vi "Wait at Rendezvous.vi"(4 "error in (no error)":errorcluster, 5 "ms timeout (-1)":i32=-1, 7 "rendezvous":T1) -> (0 "error out":errorcluster, 1 "timed out":bool, 3 "rendezvous out":T1)   [LabVIEW 2010]
doc: "Waits until a sufficient number of tasks have arrived at the rendezvous."
uses:
  RendezvousDataCluster.ctl
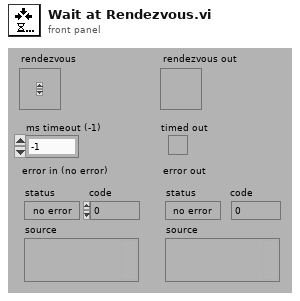
[diagram p1: front panel]
types:
  T1 = typedef "Rendezvous RefNum" = refnum<k1>
  T2 = typedef "RendezvousDataCluster.ctl" = cluster{"Threshold":i32, "Messenger Queues":refnum<queue>[]}
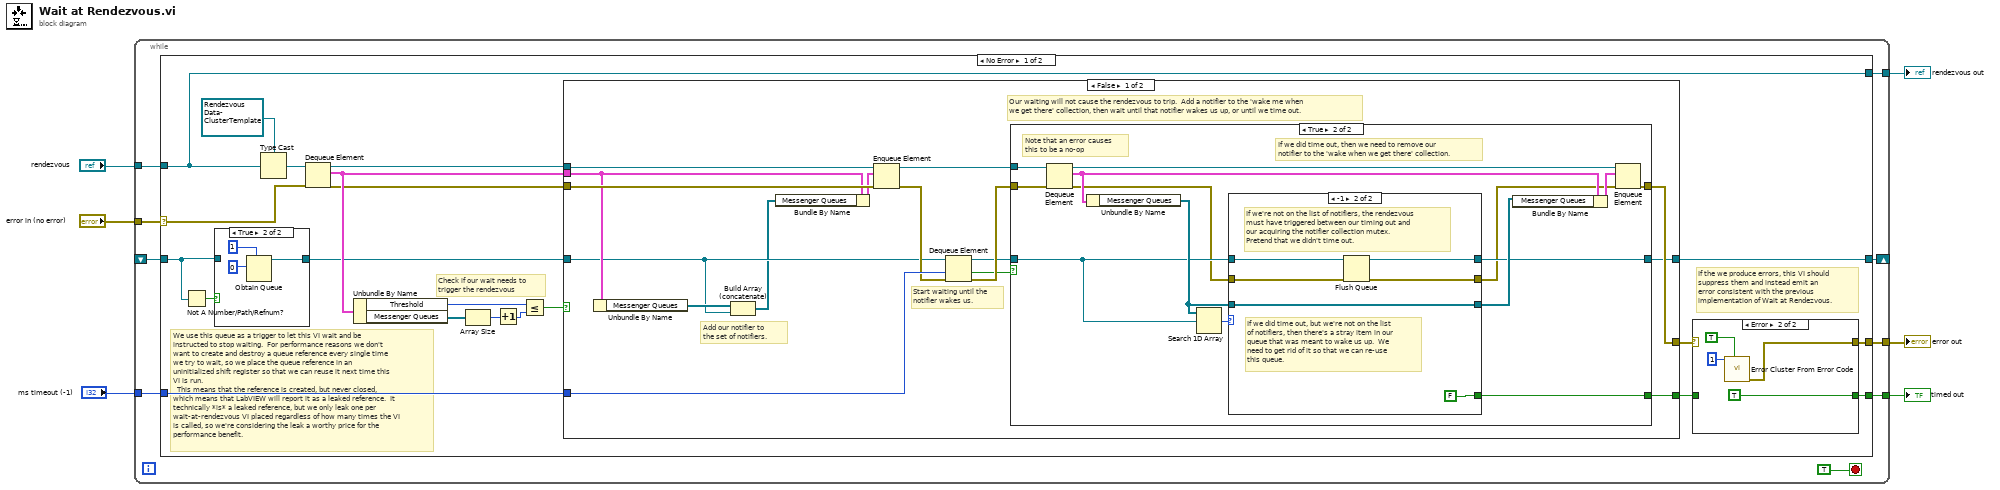
[diagram p0: block diagram]
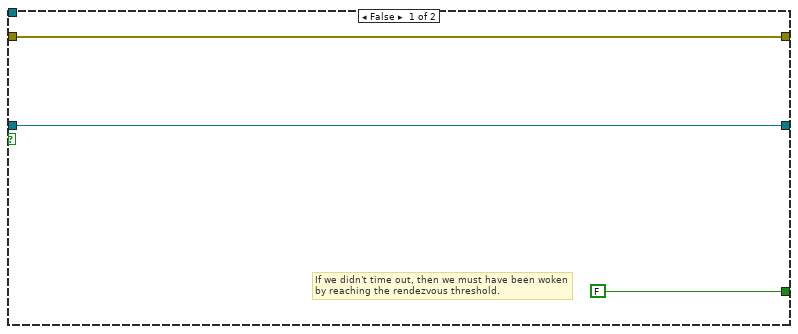
[diagram p3: hidden frame]
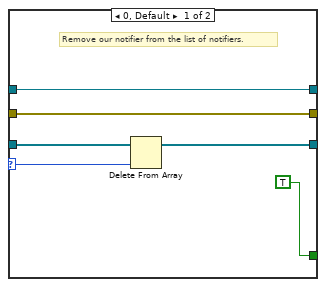
[diagram p4: hidden frame]
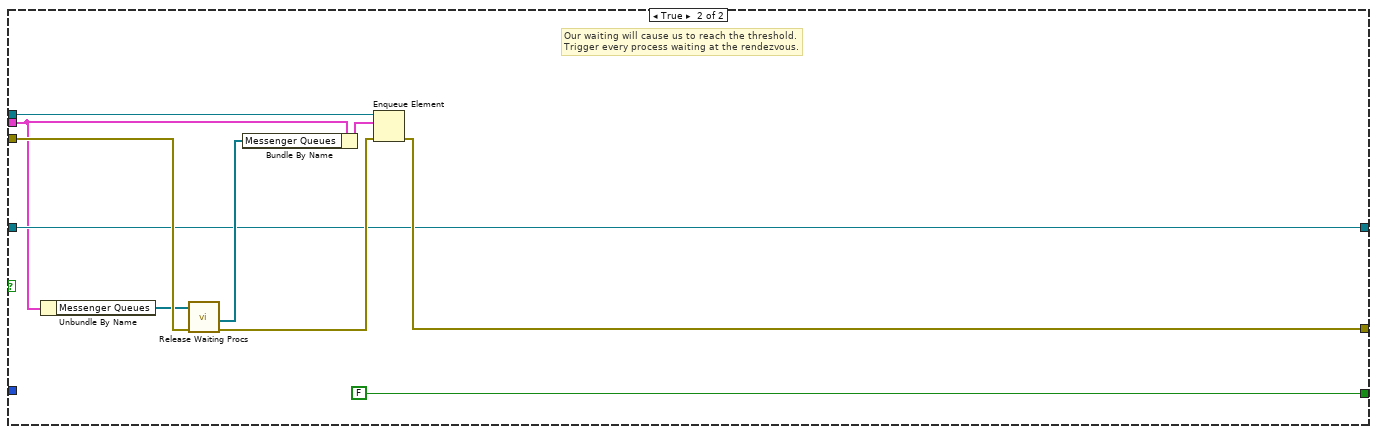
[diagram p5: hidden frame]
diagram:
  n1 = while {
    tunnel: [w15] -> w6
    tunnel: [w14] -> w5
    tunnel: "rendezvous" -> [w13]
    tunnel: [w12] -> w3
    tunnel: "error in (no error)" -> [w11]
    tunnel: "ms timeout (-1)" -> [w10]
    shift-right: [w8] -> _
    shift-left: _ -> [w7]
    stop <- TRUE stop-if-true
    n2 = case shown="No Error" w11 {
      selector: w11 -> [w23 w105]
      tunnel: [w36 w105] -> w15
      tunnel: [w35 FALSE] -> w14
      tunnel: w13 -> [w21 w104]
      tunnel: [w21 w104] -> w12
      tunnel: w10 -> [w29 _]
      tunnel: [w20 w102] -> w8
      tunnel: w7 -> [w17 w102]
      frame No Error {
        # "We use this queue as a trigger to let this VI wait and be instructed to stop waiting.  For performance reasons we don't want to create and destroy a queue reference every single time we try to wait, so we place the queue reference in an uninitialized shift register so that we can reuse it next time this VI is run.  \n  This means that the reference is created, but never closed, which means that LabVIEW will report it as a leaked reference.  It technically *is* a leaked reference, but we only leak one per wait-at-rendezvous VI placed regardless of how many times the VI is called, so we're considering the leak a worthy price for the performance benefit."
        # "Check if our wait needs to trigger the rendezvous"
        # "If the we produce errors, this VI should suppress them and instead emit an error consistent with the previous implementation of Wait at Rendezvous."
        n3 = Not A Number/Path/Refnum?(number/path/refnum=w17) -> (NaN/Path/Refnum?=w18:bool)
        n4 = case shown="True" w18 {
          tunnel: [w37 w38] -> w19
          tunnel: w17 -> [w37 _]
          frame False {
          }
          frame True {
            n5 = Obtain Queue(max queue size (-1, unlimited)=1, element data type=0) -> (queue out=w38:refnum<queue>)  [unwired: 2 in, 3 out]
          }
        }
        n6 = Type Cast(type=refnum<queue> refnum ("queue out"), x=w21) -> (*(type *) &x=w22:refnum<queue>)
        n7 = Dequeue Element(queue=w22, error in (no error)=w23) -> (queue out=w31:refnum<queue>, element=w27:T2, error out=w25:errorcluster)  [unwired: 2 out]
        n8 = Unbundle By Name(w27) -> ("Threshold"=w33:i32, "Messenger Queues"=w24:refnum<queue>[])
        n9 = Array Size(array=w24) -> (size(s)=w26:i32)
        n10 = Increment(x=w26) -> (x+1=w34:i32)
        n11 = Less Or Equal?(x=w33, y=w34) -> (x <= y?=w32:bool)
        n12 = case shown="False" w32 {
          tunnel: [w56 w93] -> w30
          tunnel: w31 -> [w54 w94]
          tunnel: w29 -> [w52 _]
          tunnel: [w55 FALSE] -> w28
          tunnel: w27 -> [w44 w86]
          tunnel: w25 -> [w53 w92]
          tunnel: [w45 w88] -> w20
          tunnel: w19 -> [w42 w88]
          frame False {
            # "Start waiting until the notifier wakes us."
            # "Add our notifier to the set of notifiers."
            # "Our waiting will not cause the rendezvous to trip.  Add a notifier to the 'wake me when we get there' collection, then wait until that notifier wakes us up, or until we time out."
            n13 = Unbundle By Name(w44) -> ("Messenger Queues"=w43:refnum<queue>[])
            n14 = Build Array (concatenate)(w43, w42) -> (w41:refnum<queue>[])
            n15 = Bundle By Name(cluster=w44, "Messenger Queues"=w41) -> (w51:T2)
            n16 = Enqueue Element(queue=w54, element=w51, error in (no error)=w53) -> (queue out=w50:refnum<queue>, error out=w49:errorcluster)  [unwired: 2 out]
            n17 = Dequeue Element(queue=w42, timeout in ms (-1)=w52, error in (no error)=w49) -> (queue out=w46:refnum<queue>, timed out?=w47:bool, error out=w48:errorcluster)  [unwired: 1 out]
            n18 = case shown="True" w47 {
              tunnel: [w58 w68] -> w56
              tunnel: [FALSE w72] -> w55
              tunnel: w50 -> [_ w71]
              tunnel: w48 -> [w58 w70]
              tunnel: w46 -> [w57 w62]
              tunnel: [w57 w63] -> w45
              frame False {
                # "If we didn't time out, then we must have been woken\nby reaching the rendezvous threshold."
              }
              frame True {
                # "Note that an error causes this to be a no-op"
                # "If we did time out, then we need to remove our notifier to the 'wake when we get there' collection."
                n19 = Dequeue Element(queue=w71, error in (no error)=w70) -> (queue out=w69:refnum<queue>, element=w66:T2, error out=w61:errorcluster)  [unwired: 2 out]
                n20 = Unbundle By Name(w66) -> ("Messenger Queues"=w67:refnum<queue>[])
                n21 = Search 1D Array(1D array=w67, element=w62) -> (index of element=w73:i32)  [unwired: 1 out]
                n22 = case shown="-1" w73 {
                  selector: w73 -> [w79 _]
                  tunnel: [w78 w84] -> w64
                  tunnel: [TRUE FALSE] -> w72
                  tunnel: w67 -> [w76 w84]
                  tunnel: [w75 w82] -> w63
                  tunnel: w62 -> [w75 w83]
                  tunnel: w61 -> [w74 w81]
                  tunnel: [w74 w80] -> w60
                  frame 0, Default {
                    # "Remove our notifier from the list of notifiers."
                    n23 = Delete From Array(array=w76, index=w79) -> (array with subset deleted=w78:refnum<queue>[])  [unwired: 1 in, 1 out]
                  }
                  frame -1 {
                    # "If we did time out, but we're not on the list of notifiers, then there's a stray item in our queue that was meant to wake us up.  We need to get rid of it so that we can re-use this queue."
                    # "If we're not on the list of notifiers, the rendezvous must have triggered between our timing out and our acquiring the notifier collection mutex.  Pretend that we didn't time out."
                    n24 = Flush Queue(queue=w83, error in (no error)=w81) -> (queue out=w82:refnum<queue>, error out=w80:errorcluster)  [unwired: 1 out]
                  }
                }
                n25 = Bundle By Name(cluster=w66, "Messenger Queues"=w64) -> (w65:T2)
                n26 = Enqueue Element(queue=w69, element=w65, error in (no error)=w60) -> (error out=w68:errorcluster)  [unwired: 3 out]
              }
            }
          }
          frame True {
            # "Our waiting will cause us to reach the threshold.\nTrigger every process waiting at the rendezvous."
            n27 = Unbundle By Name(w86) -> ("Messenger Queues"=w87:refnum<queue>[])
            n28 = call "Release Waiting Procs.vi"("error in (no error)"=w92, "Notifiers"=w87) -> ("Error Out"=w91:errorcluster, "Notifiers Out"=w89:refnum<queue>[])  [unwired: 1 in, 7 out]
            n29 = Bundle By Name(cluster=w86, "Messenger Queues"=w89) -> (w90:T2)
            n30 = Enqueue Element(queue=w94, element=w90, error in (no error)=w91) -> (error out=w93:errorcluster)  [unwired: 3 out]
          }
        }
        n31 = case shown="Error" w30 {
          selector: w30 -> [w97 _]
          tunnel: [w97 w101] -> w36
          tunnel: [w96 TRUE] -> w35
          tunnel: w28 -> [w96 _]
          frame No Error {
          }
          frame Error {
            n32 = call "Error Cluster From Error Code.vi"("show call chain? (False)"=TRUE, "error code (0)"=1) -> ("error out"=w101:errorcluster)  [unwired: 1 in, 6 out]
          }
        }
      }
      frame Error {
        # "If there was an error, do not interact\nwith the rendezvous at all."
      }
    }
  }
  "rendezvous out" <- w3
  "error out" <- w6
  "timed out" <- w5
